vi "Start Transaction.vi"(4 "error in":errorcluster, 7 "Connection In":refnum<k7>) -> (0 "error out":errorcluster, 3 "Connection Out":refnum<k7>)   [LabVIEW 2020, in "hse-db-ado.lvlib" / "ADO-DB-Driver.lvlib"]
doc: "Start a transaction\n\n____\nHAMPEL SOFTWARE ENGINEERING v1.4.0 (2023-12-19 09:52)"
uses:
  ADO-DB-Driver.lvlib
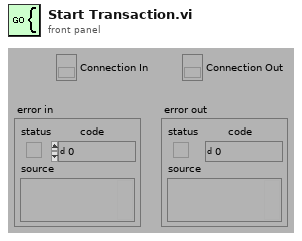
[diagram p1: front panel]
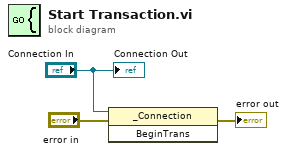
[diagram p0: block diagram]
diagram:
  n1 = invoke class="_Connection" method="BeginTrans"(reference="Connection In", error in="error in") -> (error out=→"error out":errorcluster)  [unwired: 1 in, 2 out]
  "Connection Out" <- "Connection In"
